vi "CreateTable.vi"(8 "error in (no error)":errorcluster, 11 "试验名称":string) -> (0 "error out":errorcluster)   [LabVIEW 2014]
panel:
  # "不可能创建新的数据库，因为要手动添加数据源\n只能建立一个数据库，然后建立这么几个表，在里面存储\n\n但是可以按时间建立不同的表\n\n还要创建交流通道的表"
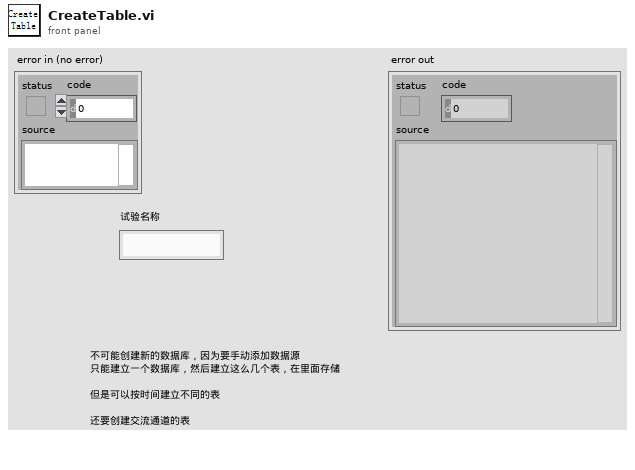
[diagram p1: front panel]
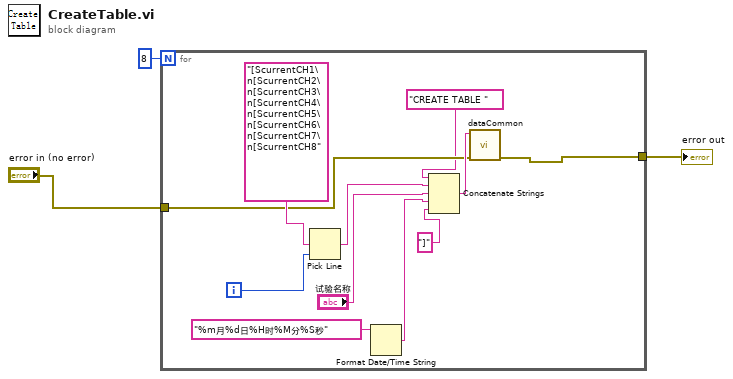
[diagram p0: block diagram]
diagram:
  n1 = for {
    N: 8 -> [_]
    tunnel: "error in (no error)" -> [w6]
    tunnel: [w5] -> w1
    i -> [w13]
    n2 = Pick Line(multi-line string="[ScurrentCH1\n[ScurrentCH2\n[ScurrentCH3\n[ScurrentCH4\n[ScurrentCH5\n[ScurrentCH6\n[ScurrentCH7\n[ScurrentCH8" ("多行字符串"), line index=w13) -> (output string=w11:string)  [unwired: 1 in]
    n3 = Format Date/Time String(time format string (%c)="%m月%d日%H时%M分%S秒" ("时间格式字符串(%c)")) -> (date/time string=w9:string)  [unwired: 2 in]
    n4 = Concatenate Strings("CREATE TABLE ", w11, "试验名称", w9, "]") -> (w7:string)
    n5 = call "dataCommon.vi"("error in (no error)"=w6, "Command Text"=w7) -> ("error out"=w5:errorcluster)  [unwired: 8 in, 1 out]
  }
  "error out" <- w1
